vi "eNames Loop.vi"() -> (0 "error out":errorcluster)   [LabVIEW 2020]
panel:
  out "Iteration":u32
  in  "Write/Read":i32[](array[ring])=[0, 0, 1, 1] items=["Read", "Write"]
  out "Values Out":dbl[][](array[numeric]) format="%.6f"
  in  "Values In":dbl[][](array[numeric])=[[0.0], [0.0], [2.34], [1.0]] format="%.3f"
  in  "NumValues":u16[](array[numeric])=[1, 1, 1, 1]
  in  "Names":string[](array[string])=["AIN0", "FIO2", "DAC0", "FIO1"]
  in  "stop":bool
  in  "Interval [ms]":i32=500
  out "Error String":string
  out "ConnectionType Out":i32
  out "DeviceType Out":i32
  in  "Identifier":string="LJM_idANY"
  in  "ConnectionType":string="LJM_ctANY"
  in  "DeviceType":string="LJM_dtANY"
  # "\"eNames Loop.vi\" and \"Read Write Loop with Config\"\nshow 2 different ways to do reads and writes\nin a loop.  Using eNames results in a single low-level\npacket, and thus is very efficient, but all the arrays can\nseem a little complex to some.  Using eReadNames and\neWriteNames results in a low-level packet for each, but\nmight seem simpler.  In fact, eAddresses is the most\nefficient because it uses 1 low-level packet and LJM\ndoes not have to convert names to addresses each\ntime in the loop (see it used in C-R Speed Test.vi)."
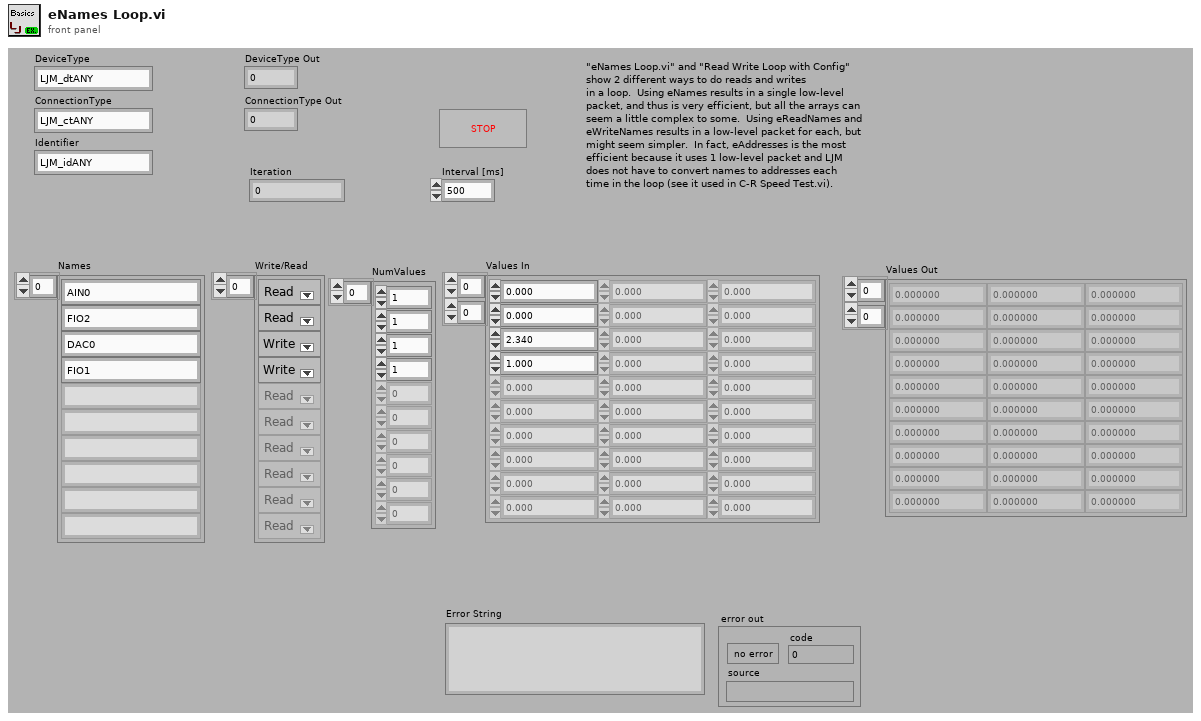
[diagram p1: front panel]
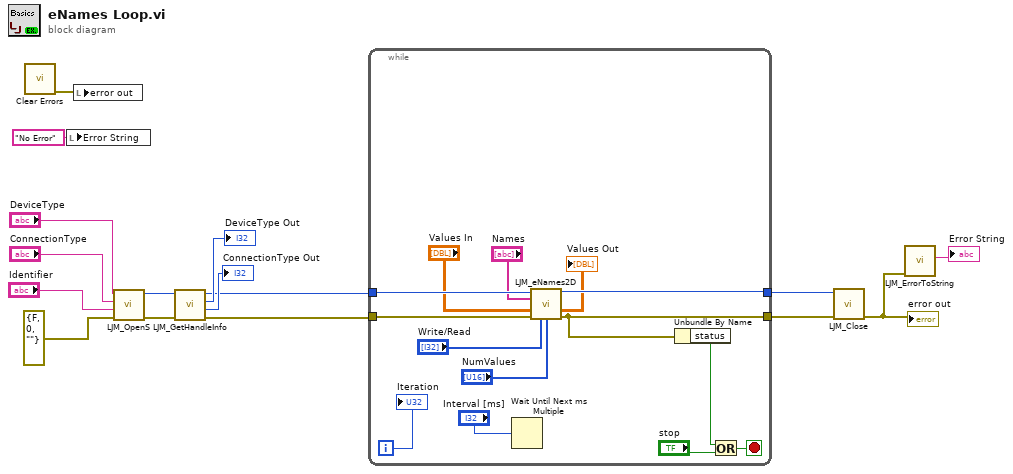
[diagram p0: block diagram]
diagram:
  n1 = call <vilib>:"Clear Errors.vi"() -> ("error out"=w2:errorcluster)  [unwired: 6 in, 1 out]
  n2 = local write "Error String"("No Error" ("Error String")) -> ()
  n3 = local write "error out"(w2) -> ()
  n4 = call "LJM_OpenS.vi"("error in"=errorcluster {"status"=FALSE, "code"=0, "source"=""}, "Identifier"="Identifier", "ConnectionType"="ConnectionType", "DeviceType"="DeviceType") -> ("error out"=w16:errorcluster, "Handle"=w15:i32)  [unwired: 6 in]
  n5 = call "LJM_GetHandleInfo.vi"("error in"=w16, "Handle In"=w15) -> ("error out"=w4:errorcluster, "ConnectionType"=→"ConnectionType Out":i32, "DeviceType"=→"DeviceType Out":i32, "Handle Out"=w5:i32)  [unwired: 2 in, 4 out]
  n6 = while {
    tunnel: w4 -> [w30]
    tunnel: [w24] -> w7
    tunnel: w5 -> [w29]
    tunnel: [w23] -> w6
    i -> [w17]
    stop <- w27 stop-if-true
    n7 = Wait Until Next ms Multiple(millisecond multiple="Interval [ms]") -> ()  [unwired: 1 out]
    n8 = call "LJM_eNames2D.vi"("Handle In"=w29, "aNames"="Names", "aValuesIn"="Values In", "error in"=w30, "aWrites"="Write/Read", "aNumValues"="NumValues") -> ("Handle Out"=w23:i32, "aValuesOut"=→"Values Out":dbl[][], "error out"=w24:errorcluster)  [unwired: 6 in, 1 out]
    n9 = Unbundle By Name(w24) -> ("status"=w26:bool)
    n10 = Or(x=w26, y="stop") -> (x .or. y?=w27:bool)
    "Iteration" <- w17
  }
  n11 = call "LJM_Close.vi"("error in"=w7, "Handle"=w6) -> ("error out"=w9:errorcluster)  [unwired: 9 in]
  "error out" <- w9
  n12 = call "LJM_ErrorToString.vi"("error in"=w9) -> ("String"=→"Error String":string)  [unwired: 10 in]
